vi "Gate.vi"() -> ()   [LabVIEW 2018]
panel:
  out "o 6":bool
  in  "y 5":bool
  in  "x 6":bool
  out "o 5":bool
  in  "y 4":bool
  in  "x 5":bool
  out "o 4":bool
  in  "x 4":bool
  out "o 3":bool
  in  "y 3":bool
  in  "x 3":bool
  out "o 2":bool
  in  "y 2":bool
  in  "x 2":bool
  out "o":bool
  in  "y":bool
  in  "x":bool
  # "OR GATE"
  # "EXOR GATE"
  # "AND GATE"
  # "NOR GATE"
  # "NAND GATE"
  # "NOT GATE"
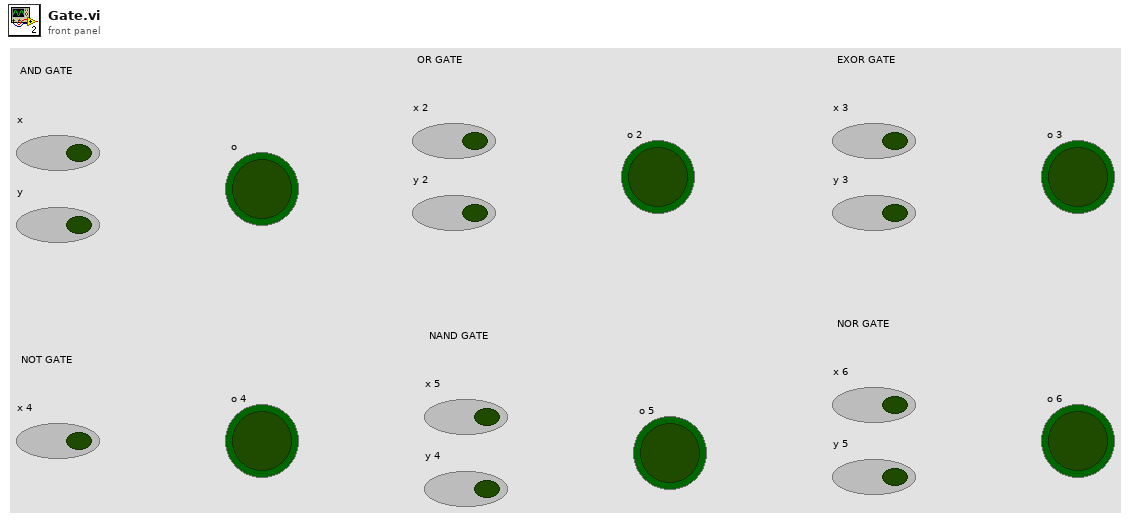
[diagram p1: front panel]
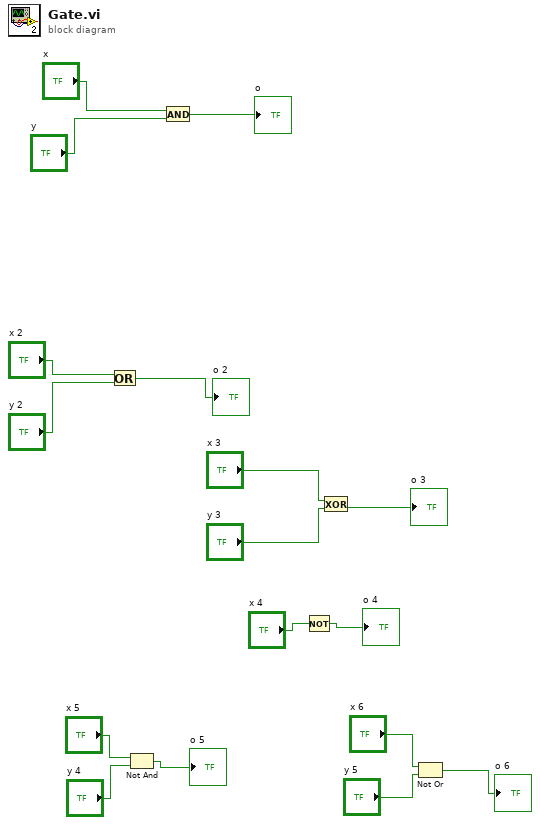
[diagram p0: block diagram]
diagram:
  n1 = Or(x="x 2", y="y 2") -> (x .or. y?=→"o 2":bool)
  n2 = Not And(1:"y 4", 2:"x 5") -> (0:→"o 5":bool)
  n3 = And(x="x", y="y") -> (x .and. y?=→"o":bool)
  n4 = Not(x="x 4") -> (.not. x?=→"o 4":bool)
  n5 = Exclusive Or(1:"y 3", 2:"x 3") -> (0:→"o 3":bool)
  n6 = Not Or(1:"y 5", 2:"x 6") -> (0:→"o 6":bool)
